vi "Get Tunnels.vi"(8 "error in (no error)":errorcluster, 11 "CSM-Helper in":refnum<class "CSM-Helper.lvclass">) -> (0 "error out":errorcluster, 3 "CSM-Helper out":refnum<class "CSM-Helper.lvclass">)   [LabVIEW 2020, in "CSM-Helper.lvclass"]
uses:
  CSM-Helper.lvclass
  CSM-Helper.lvclass/CSM-Helper.ctl
  <vilib>/Utility/Data Type/Type Definitions/Data Type.ctl
  <vilib>/Utility/Data Type/Type Definitions/Refnum Type.ctl
  <vilib>/Utility/Data Type/NI_Data Type.lvlib
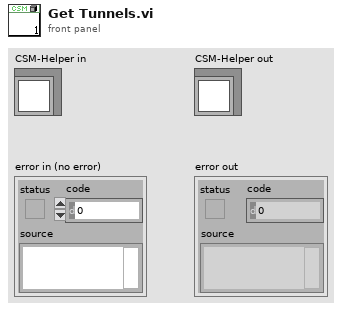
[diagram p1: front panel]
types:
  T1 = cluster{refnum<vi>, "Outer Term":refnum<vi>, "Data Type":variant, "Wire":refnum<vi>}
  T2 = typedef "NI_Data Type.lvlib/Data Type.ctl" = enum8{"Invalid Type", "Void", "I8", "I16", "I32", "I64", "U8", "U16", "U32", "U64", "Single Float", "Double Float", "Extended Float", "Single Complex", "Double Complex", "Extended Complex", "Enum U8", "Enum U16", "Enum U32", "Enum U64", "Single Float With Unit", "Double Float With Unit", "Extended Float With Unit", "Single Complex with Unit", "Double Complex with Unit", "Extended Complex with Unit", "Boolean", "String", "Path", "Picture", "Tag", "Array", "Cluster", "Variant", "LV Variant", "Waveform", "Timestamp", "Digital Waveform", "Digital Data", "ExpressData", "Refnum", "External Data", "VI", "Poly VI", "LabVIEW Class Instance", "Fixed Point", "Set Collection", "Map Collection"}
  T3 = typedef "NI_Data Type.lvlib/Type Definition Info.ctl" = cluster{"Name":string, "Timestamp":u32}
  T4 = typedef "NI_Data Type.lvlib/Refnum Type.ctl" = enum16{"NotARefnum", "UnknownRefnum", "Generic", "Datalog", "ByteStream", "Device", "Occurence", "TCPNetConnection", "Auto", "Menu", "Imaq", "Hardware", "DataSocket", "Visa", "IVI", "UDPNetConnection", "Notifier", "Queue", "Irda", "EventReg", "DotNet", "UserEvent", "Callback", "UNUSED_EMPTY_POSITION", "BlueToothNetConnection", "LVObjApp", "LVObjVI", "LVObjUnknown", "GenericClass", "UserDefinedRefnumTag", "DataValue", "RT FIFO", "TDMS File", "PythonSessionRefnum"}
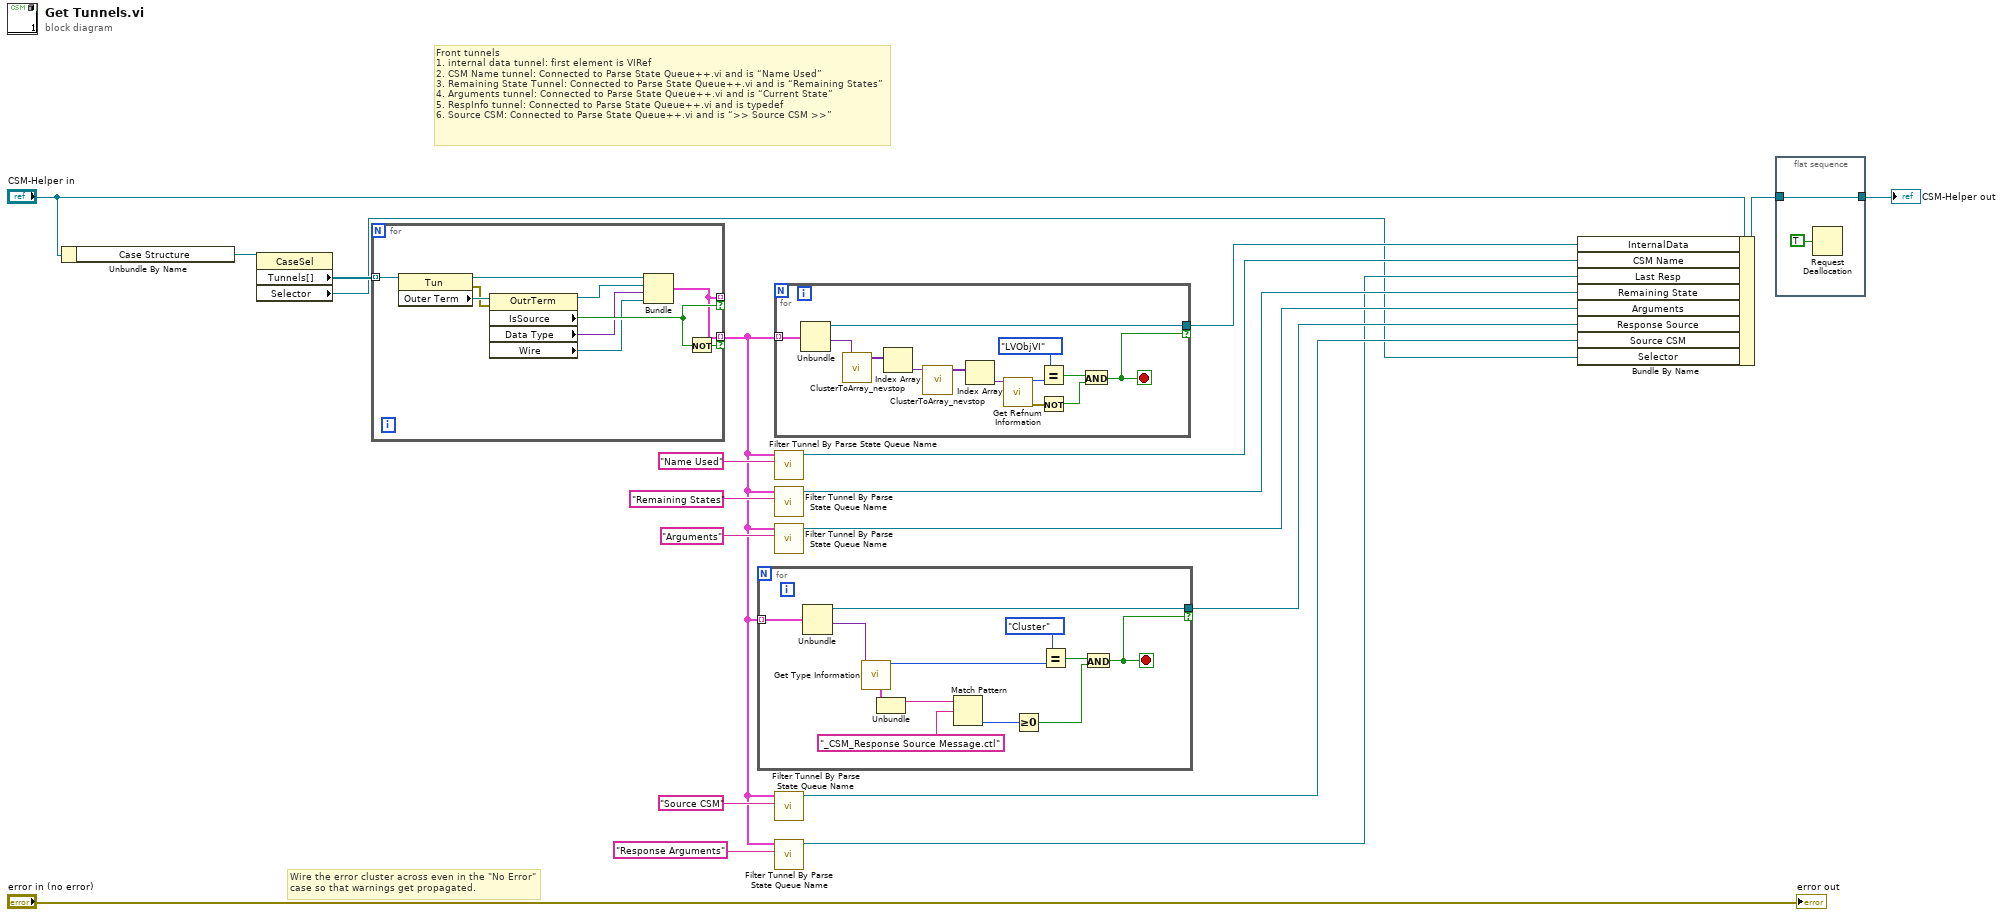
[diagram p0: block diagram]
diagram:
  # "Front tunnels\n1. internal data tunnel: first element is VIRef\n2. CSM Name tunnel: Connected to Parse State Queue++.vi and is “Name Used”\n3. Remaining State Tunnel: Connected to Parse State Queue++.vi and is “Remaining States”\n4. Arguments tunnel: Connected to Parse State Queue++.vi and is “Current State”\n5. RespInfo tunnel: Connected to Parse State Queue++.vi and is typedef\n6. Source CSM: Connected to Parse State Queue++.vi and is “>> Source CSM >>”"
  # "Wire the error cluster across even in the \"No Error\"\ncase so that warnings get propagated."
  n1 = Unbundle By Name("CSM-Helper in") -> ("Case Structure"=w18:refnum<vi>)
  n2 = property class="CaseSel"(reference=w18) -> ("Tunnels[]"=w17:refnum<vi>[], "Selector"=w3:refnum<vi>)  [unwired: 1 in, 2 out]
  n3 = for {
    tunnel: w17 -> [w30] mode=indexing
    tunnel: [w23] -> _ mode=indexing if=w27
    tunnel: [w23] -> w6 mode=indexing if=w26
    n4 = property class="Tun"(reference=w30) -> (reference out=w25:refnum<vi>, error out=w28:errorcluster, "Outer Term"=w29:refnum<vi>)  [unwired: 1 in]
    n5 = property class="OutrTerm"(reference=w29, error in=w28) -> (reference out=w24:refnum<vi>, "IsSource"=w27:bool, "Data Type"=w22:variant, "Wire"=w21:refnum<vi>)  [unwired: 1 out]
    n6 = Bundle(w25, "Outer Term"=w24, "Data Type"=w22, "Wire"=w21) -> (w23:T1)  [unwired: 1 in]
    n7 = Not(x=w27) -> (.not. x?=w26:bool)
  }
  n8 = for {
    tunnel: w6 -> [w42] mode=indexing
    tunnel: [w39] -> w7 if=w38
    stop <- w38 stop-if-true
    n9 = Unbundle(w42) -> (w39:refnum<vi>, "Data Type"=w35:variant)  [unwired: 2 out]
    n10 = call <vilib>:"Get Type Information.vi"("variant"=w35) -> ("type"=w41:T2, "type definition info"=w36:T3)  [unwired: 6 in, 3 out]
    n11 = Unbundle(w36) -> ("Name"=w34:string)  [unwired: 1 out]
    n12 = Match Pattern(string=w34, regular expression="_CSM_Response Source Message.ctl") -> (offset past match=w32:i32)  [unwired: 1 in, 3 out]
    n13 = Greater Or Equal To 0?(x=w32) -> (x >= 0?=w31:bool)
    n14 = Equal?(x=Data_Type."Cluster", y=w41) -> (x = y?=w40:bool)
    n15 = And(x=w40, y=w31) -> (x .and. y?=w38:bool)
  }
  n16 = for {
    tunnel: w6 -> [w55] mode=indexing
    tunnel: [w44] -> w16 if=w43
    stop <- w43 stop-if-true
    n17 = Unbundle(w55) -> (w44:refnum<vi>, "Data Type"=w54:variant)  [unwired: 2 out]
    n18 = call <userlib>:"ClusterToArray_nevstop.vi"("Cluster"=w54) -> ("Array"=w53:variant[])  [unwired: 10 in]
    n19 = Index Array(array=w53) -> (element=w52:variant)  [unwired: 1 in]
    n20 = call <userlib>:"ClusterToArray_nevstop.vi"("Cluster"=w52) -> ("Array"=w51:variant[])  [unwired: 10 in]
    n21 = Index Array(array=w51) -> (element=w50:variant)  [unwired: 1 in]
    n22 = call <vilib>:"Get Refnum Information.vi"("variant"=w50) -> ("error out"=w46:errorcluster, "reference type"=w48:T4)  [unwired: 7 in, 2 out]
    n23 = Equal?(x=Refnum_Type."LVObjVI", y=w48) -> (x = y?=w47:bool)
    n24 = Not(x=w46) -> (.not. x?=w45:bool)
    n25 = And(x=w47, y=w45) -> (x .and. y?=w43:bool)
  }
  n26 = call "Filter Tunnel By Parse State Queue Name.vi"("regular expression"="Name Used", "Array"=w6) -> ("Tunnel out"=w15:refnum<vi>)  [unwired: 9 in]
  n27 = call "Filter Tunnel By Parse State Queue Name.vi"("regular expression"="Remaining States", "Array"=w6) -> ("Tunnel out"=w12:refnum<vi>)  [unwired: 9 in]
  n28 = call "Filter Tunnel By Parse State Queue Name.vi"("regular expression"="Arguments", "Array"=w6) -> ("Tunnel out"=w10:refnum<vi>)  [unwired: 9 in]
  n29 = call "Filter Tunnel By Parse State Queue Name.vi"("regular expression"="Source CSM", "Array"=w6) -> ("Tunnel out"=w8:refnum<vi>)  [unwired: 9 in]
  n30 = call "Filter Tunnel By Parse State Queue Name.vi"("regular expression"="Response Arguments", "Array"=w6) -> ("Tunnel out"=w4:refnum<vi>)  [unwired: 9 in]
  n31 = Bundle By Name(cluster="CSM-Helper in", "InternalData"=w16, "CSM Name"=w15, "Last Resp"=w4, "Remaining State"=w12, "Arguments"=w10, "Response Source"=w7, "Source CSM"=w8, "Selector"=w3) -> (w2:refnum<class "CSM-Helper.lvclass">)
  n32 = flat-sequence {
    tunnel: w2 -> [w56]
    tunnel: [w56] -> w1
    frame #0 {
      n33 = Request Deallocation(TRUE ("flag")) -> ()
    }
  }
  "error out" <- "error in (no error)"
  "CSM-Helper out" <- w1
